vi "ALTS-2015 Extract Test Data from Array.vi"(8 "error in":errorcluster, 10 "data":string[][](array[string]), 11 "Station Enum":T1) -> (0 "error out":errorcluster, 3 "Test Result":string)   [LabVIEW 2013]
doc: "Copyright © 2005, Soliton Technologies.\nAll rights reserved."
uses:
  Controls/ALTS-2015 Station Details.ctl
  Controls/ALTS-2015 Status Ring Indicator.ctl
  Controls/ALTS-2015 Station Cluster.ctl
  Controls/ALTS-2015 LV2GBL Station Info Options.ctl
  Controls/ALTS-2015 Ring Indicator Enum.ctl
panel:
  in  "Station":T2
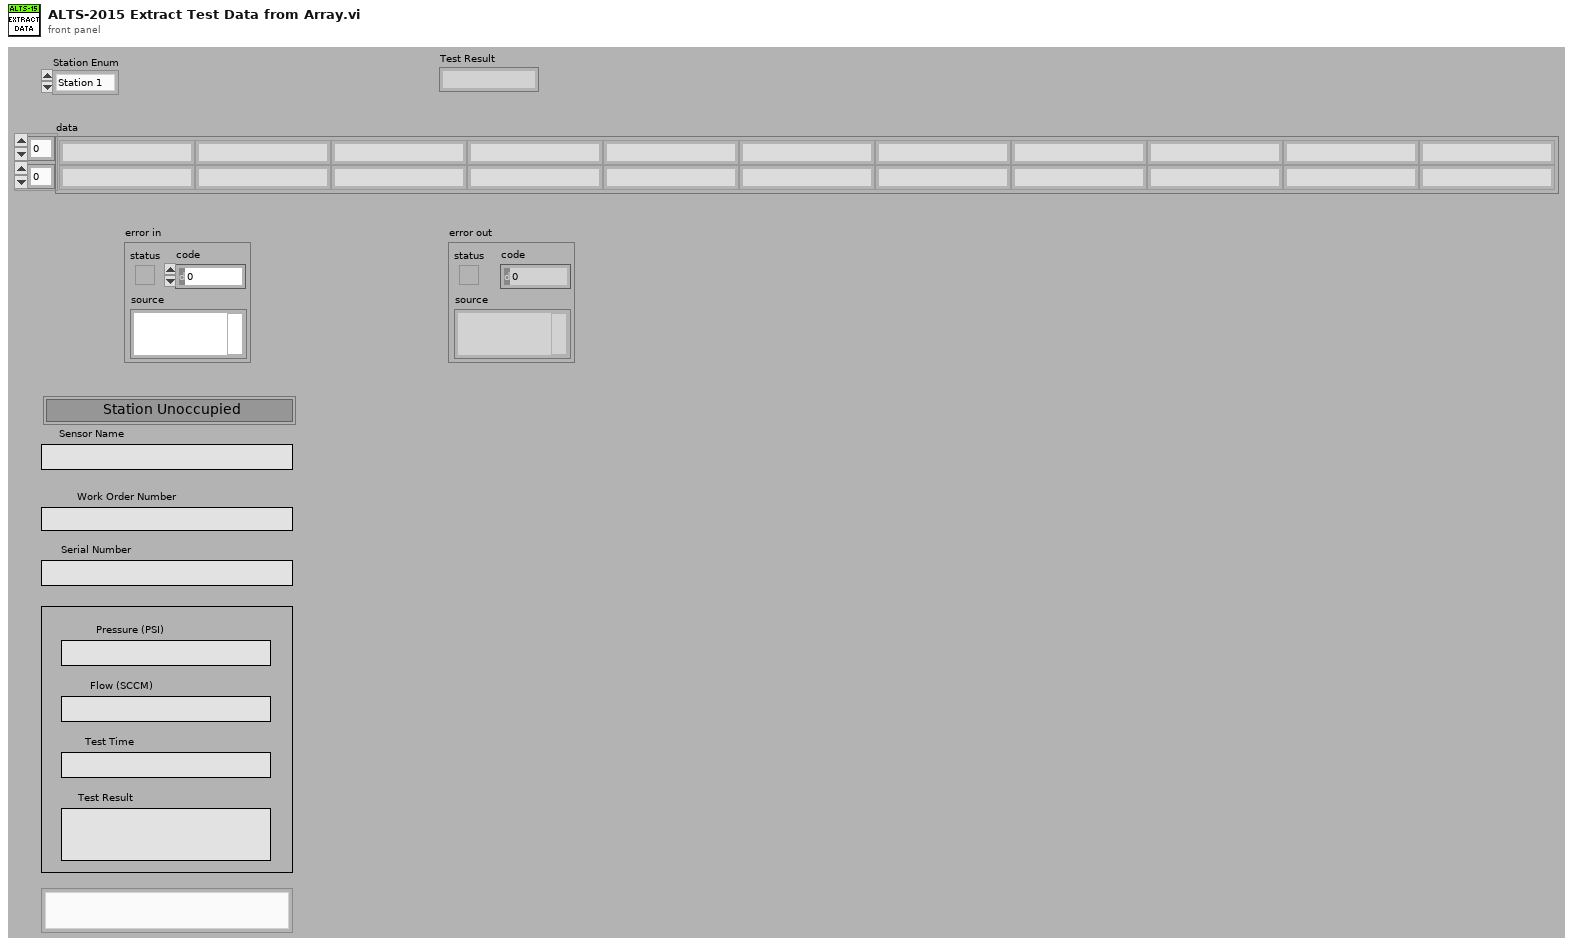
[diagram p1: front panel]
types:
  T1 = typedef "ALTS-2015 Station Cluster.ctl" = enum16{"Station 1", "Station 2", "Station 3", "Station 4"}
  T2 = typedef "ALTS-2015 Station Details.ctl" = cluster{"Station Number":string, "Work Order Number":string, "Sensor Name":string, "Pressure (PSI)":string, "Flow (SCCM)":string, "Test Time ":string, "Test Result":string, "Serial Number":string, "Station Status":T3, "Station Occupied?":bool, "Rerun Count":i32, "Test Type":i32}
  T3 = typedef "ALTS-2015 Status Ring Indicator.ctl" = u16
  T4 = typedef "ALTS-2015 Ring Indicator Enum.ctl" = enum16{"Idle", "Test Running", "Unit Clamped", "Unit not Clamped", "Pass", "Fail"}
  T5 = typedef "ALTS-2015 LV2GBL Station Info Options.ctl" = enum16{"Init", "Read", "Read All", "Write Sensor ID", "Write  WO & SN", "Write Test Data", "Write Station Status", "Write Station Occupancy", "Write Rerun", "Clear All", "Clear Test Result"}
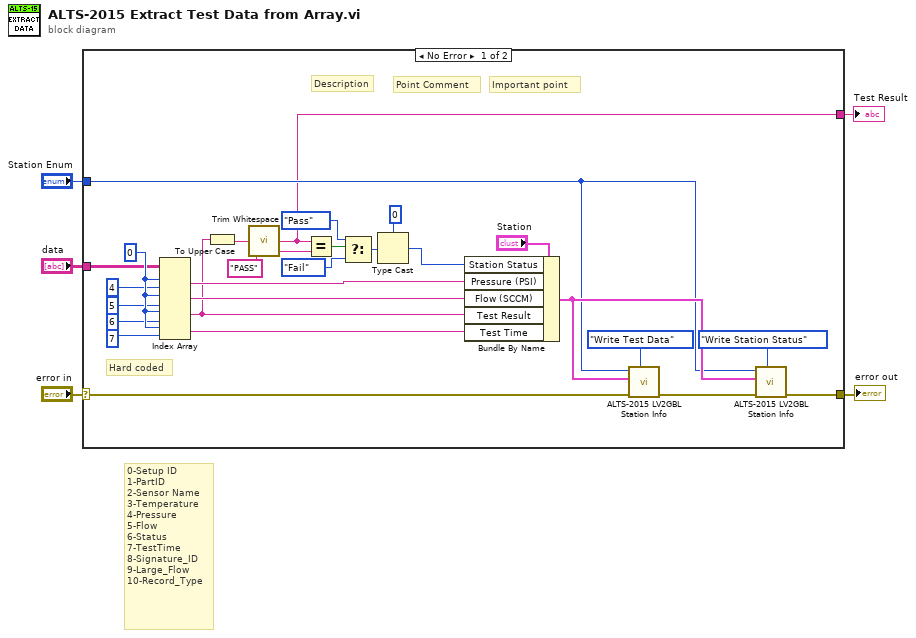
[diagram p0: block diagram]
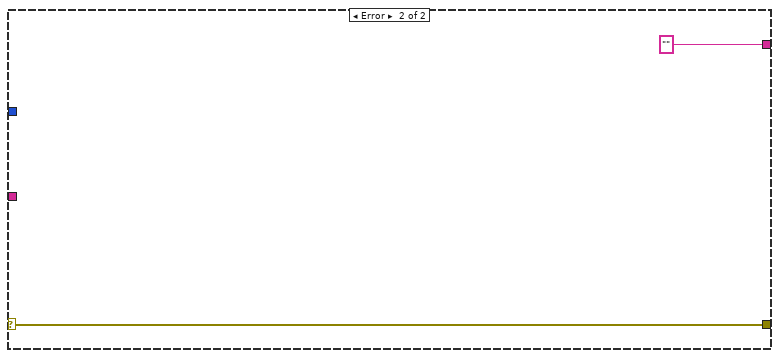
[diagram p2: hidden frame]
diagram:
  # "0-Setup ID\n1-PartID\n2-Sensor Name\n3-Temperature\n4-Pressure\n5-Flow\n6-Status\n7-TestTime\n8-Signature_ID\n9-Large_Flow\n10-Record_Type"
  n1 = case shown="No Error" "error in" {
    selector: "error in" -> [w28 w34]
    tunnel: [w29 w34] -> w4
    tunnel: "data" -> [w23 _]
    tunnel: "Station Enum" -> [w15 _]
    tunnel: [w6 "" ("Sensor Name 4")] -> w1
    frame No Error {
      w27 = 0 ("index (row)")
      # "Hard coded"
      # "Point Comment"
      # "Important point"
      # "Description"
      n2 = Index Array(array=w23, index (row) #1=w27, index (col) #1=4 ("disabled index (col)"), index (row) #2=w27, index (col) #2=5 ("disabled index (col)"), index (row) #3=w27, index (col) #3=6 ("disabled index (col)"), index (row) #4=w27, index (col) #4=7 ("disabled index (col)")) -> (element #1=w19:string, element #2=w20:string, element #3=w13:string, element #4=w14:string)
      n3 = To Upper Case(1:w13) -> (0:w7:string)
      n4 = call <vilib>:"Trim Whitespace.vi"("string"=w7) -> ("trimmed string"=w6:string)  [unwired: 1 in]
      n5 = Equal?(x=w6, y="PASS") -> (x = y?=w17:bool)
      n6 = Select(t=ALTS-2015_Ring_Indicator_Enum."Pass" ("Ring Indicator Options"), s=w17, f=ALTS-2015_Ring_Indicator_Enum."Fail" ("Ring Indicator Options")) -> (s? t:f=w9:T4)
      n7 = Type Cast(type=T3 0 ("Station Status"), x=w9) -> (*(type *) &x=w8:T3)
      n8 = Bundle By Name(cluster="Station", "Station Status"=w8, "Pressure (PSI)"=w19, "Flow (SCCM)"=w20, "Test Result"=w13, "Test Time"=w14) -> (w16:T2)
      n9 = call "ALTS-2015 LV2GBL Station Info.vi"("Options"=ALTS-2015_LV2GBL_Station_Info_Options."Write Test Data", "error in"=w28, "Station"=w16, "Station Cluster"=w15) -> ("error out"=w30:errorcluster)  [unwired: 5 in, 2 out]
      n10 = call "ALTS-2015 LV2GBL Station Info.vi"("Options"=ALTS-2015_LV2GBL_Station_Info_Options."Write Station Status", "error in"=w30, "Station"=w16, "Station Cluster"=w15) -> ("error out"=w29:errorcluster)  [unwired: 5 in, 2 out]
    }
    frame Error {
    }
  }
  "error out" <- w4
  "Test Result" <- w1
